vi "Coerce Experiment Inputs.vi"(8 "Error In":errorcluster, 10 "Experiment Inputs":T1) -> (0 "Error Out":errorcluster, 2 "Experiment Inputs Out":T1)   [LabVIEW 2015]
uses:
  Controls/Signal Type.ctl
  Controls/Experiment Inputs.ctl
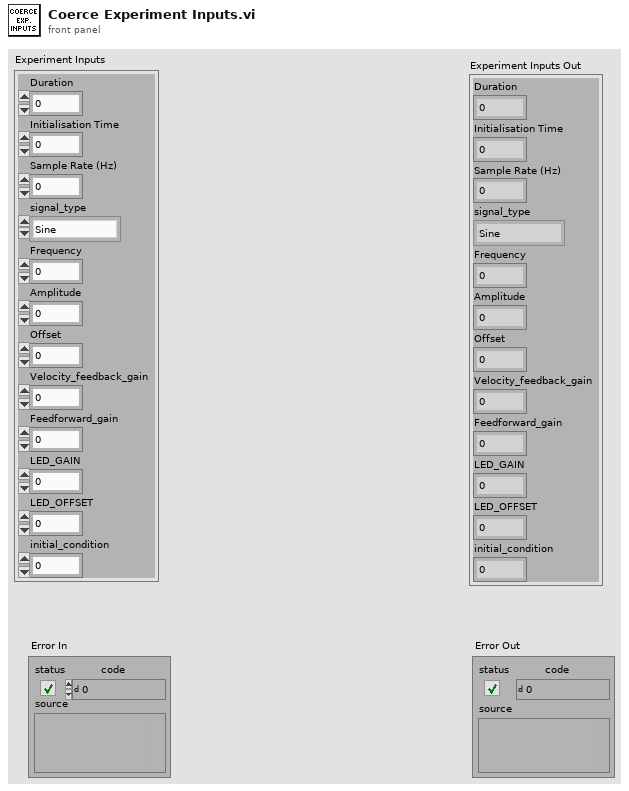
[diagram p1: front panel]
types:
  T1 = typedef "Experiment Inputs.ctl" = cluster{"Duration":dbl, "Initialisation Time":dbl, "Sample Rate (Hz)":dbl, "signal_type":T2, "Frequency":dbl, "Amplitude":dbl, "Offset":dbl, "Velocity_feedback_gain":dbl, "Feedforward_gain":dbl, "LED_GAIN":dbl, "LED_OFFSET":dbl, "initial_condition":dbl}
  T2 = typedef "Signal Type.ctl" = enum16{"Sine", "Cosine", "Square", "Step"}
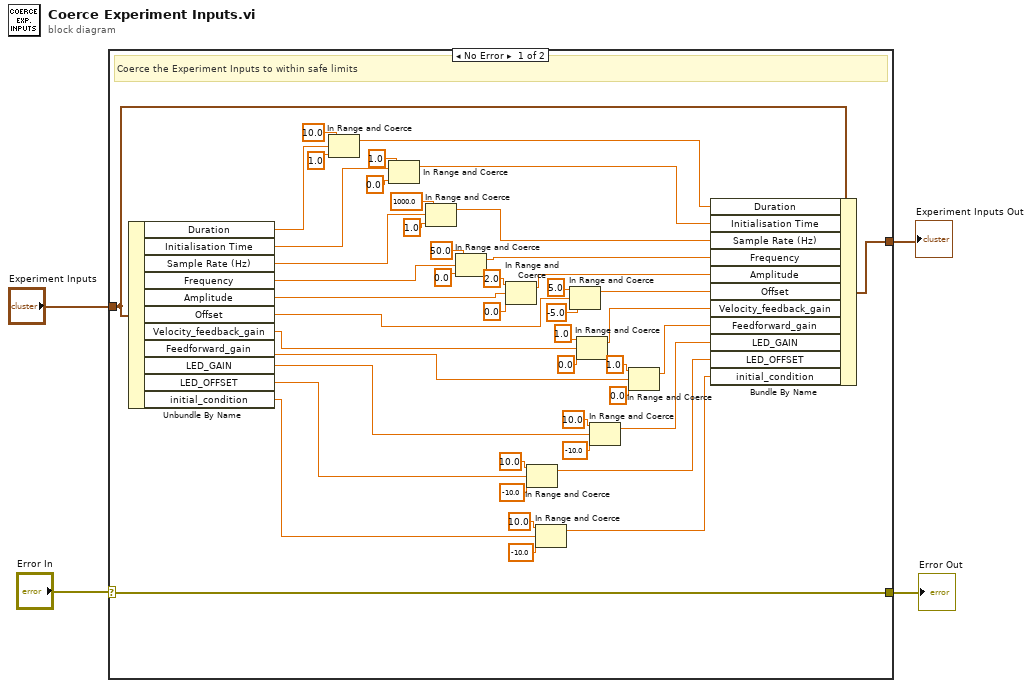
[diagram p0: block diagram]
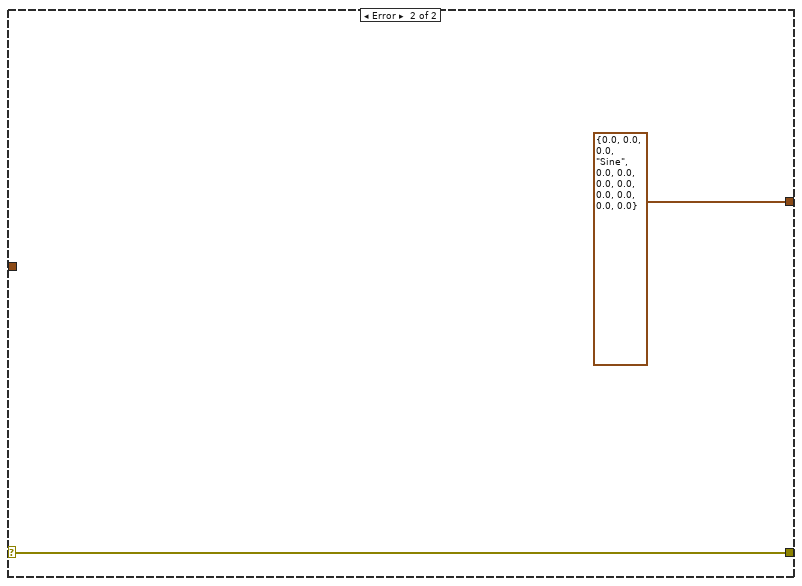
[diagram p2: hidden frame]
diagram:
  n1 = case shown="No Error" "Error In" {
    selector: "Error In" -> [w51 w52]
    tunnel: [w51 w52] -> w3
    tunnel: "Experiment Inputs" -> [w47 _]
    tunnel: [w30 T1 {"Duration"=0.0, "Initialisation Time"=0.0, "Sample Rate (Hz)"=0.0, "signal_type"=enum."Sine", "Frequency"=0.0, "Amplitude"=0.0, "Offset"=0.0, "Velocity_feedback_gain"=0.0, "Feedforward_gain"=0.0, "LED_GAIN"=0.0, "LED_OFFSET"=0.0, "initial_condition"=0.0} ("Experiment Inputs")] -> w1
    frame No Error {
      # "Coerce the Experiment Inputs to within safe limits"
      n2 = Unbundle By Name(w47) -> ("Duration"=w50:dbl, "Initialisation Time"=w43:dbl, "Sample Rate (Hz)"=w11:dbl, "Frequency"=w39:dbl, "Amplitude"=w37:dbl, "Offset"=w8:dbl, "Velocity_feedback_gain"=w33:dbl, "Feedforward_gain"=w26:dbl, "LED_GAIN"=w23:dbl, "LED_OFFSET"=w19:dbl, "initial_condition"=w15:dbl)
      n3 = In Range and Coerce(upper limit=10.0, x=w50, lower limit=1.0) -> (coerced(x)=w46:dbl)  [unwired: 1 out]
      n4 = In Range and Coerce(upper limit=1.0, x=w43, lower limit=0.0) -> (coerced(x)=w42:dbl)  [unwired: 1 out]
      n5 = In Range and Coerce(upper limit=1000.0, x=w11, lower limit=1.0) -> (coerced(x)=w10:dbl)  [unwired: 1 out]
      n6 = In Range and Coerce(upper limit=50.0, x=w39, lower limit=0.0) -> (coerced(x)=w38:dbl)  [unwired: 1 out]
      n7 = In Range and Coerce(upper limit=2.0, x=w37, lower limit=0.0) -> (coerced(x)=w32:dbl)  [unwired: 1 out]
      n8 = In Range and Coerce(upper limit=10.0, x=w19, lower limit=-10.0) -> (coerced(x)=w18:dbl)  [unwired: 1 out]
      n9 = In Range and Coerce(upper limit=10.0, x=w15, lower limit=-10.0) -> (coerced(x)=w14:dbl)  [unwired: 1 out]
      n10 = In Range and Coerce(upper limit=5.0, x=w8, lower limit=-5.0) -> (coerced(x)=w6:dbl)  [unwired: 1 out]
      n11 = In Range and Coerce(upper limit=1.0, x=w33, lower limit=0.0) -> (coerced(x)=w31:dbl)  [unwired: 1 out]
      n12 = In Range and Coerce(upper limit=10.0, x=w23, lower limit=-10.0) -> (coerced(x)=w22:dbl)  [unwired: 1 out]
      n13 = In Range and Coerce(upper limit=1.0, x=w26, lower limit=0.0) -> (coerced(x)=w27:dbl)  [unwired: 1 out]
      n14 = Bundle By Name(cluster=w47, "Duration"=w46, "Initialisation Time"=w42, "Sample Rate (Hz)"=w10, "Frequency"=w38, "Amplitude"=w32, "Offset"=w6, "Velocity_feedback_gain"=w31, "Feedforward_gain"=w27, "LED_GAIN"=w22, "LED_OFFSET"=w18, "initial_condition"=w14) -> (w30:T1)
    }
    frame Error {
    }
  }
  "Error Out" <- w3
  "Experiment Inputs Out" <- w1
